vi "FlexDDS-NG_DCP_Command_bool.vi"(8 "Write DCP command?":bool=TRUE, 9 "command string":string="update:u", 10 "Channels":T1(ring)=enum."Both channels", 11 "initial instruction string":string) -> (3 "appended instruction string":string="dcp update:u\r")   [LabVIEW 2016]
panel:
  # "Send raw 48 bit instruction"
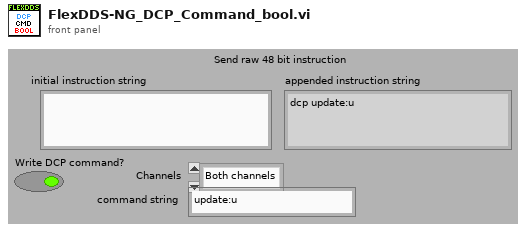
[diagram p1: front panel]
types:
  T1 = enum32{"Channel 0", "Channel 1", "Both channels"}
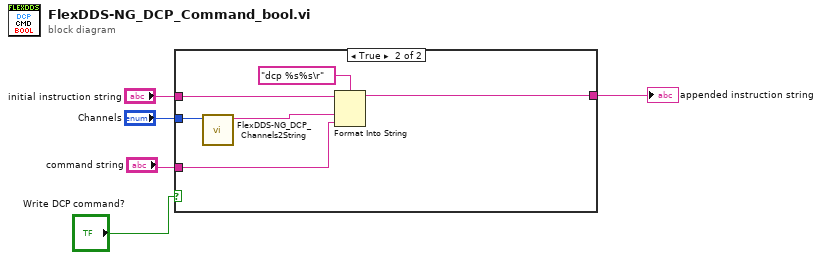
[diagram p0: block diagram]
diagram:
  n1 = case shown="True" "Write DCP command?" {
    tunnel: "initial instruction string" -> [w6 w12]
    tunnel: "Channels" -> [_ w10]
    tunnel: "command string" -> [_ w8]
    tunnel: [w6 w7] -> w2
    frame False {
    }
    frame True {
      n2 = call "FlexDDS-NG_DCP_Channels2String.vi"("Channels"=w10) -> ("channels string"=w9:string)  [unwired: 10 in]
      n3 = Format Into String(format string="dcp %s%s\r", initial string=w12, w9, w8) -> (resulting string=w7:string)  [unwired: 1 in, 1 out]
    }
  }
  "appended instruction string" <- w2
